vi "ISEG_HVSystem.constructor.vi"(0 "name":string, 2 "data in":string, 5 "error in (no error)":errorcluster) -> (14 "i ref out":refnum<vi>, 16 "data out":string, 19 "error out":errorcluster)   [LabVIEW 2014, in "ISEG_HVSystem.lvlib"]
doc: "This is the constructor of a class.\n\nLicense Agreement for this software:\n\nCopyright (C)\nGesellschaft für Schwerionenforschung, GSI\nPlanckstr. 1\n64291 Darmstadt\nGermany\n\nContact: D.Beck@gsi.de \n\nThis program is free software; you can redistribute it and/or modify it under the terms of the \nGNU General Public License as published by the Free Software Foundation; either version 2 of \nthe license, or (at your option) any later version.\n\nThis program is distributed in the hope that it will be useful, but WITHOUT ANY WARRANTY; \nwithout even the implied warranty of MERCHANTABILITY or FITNESS FOR A PARTICULAR PURPOSE. See the GNU General License for more details (http://www.gnu.org).\n\nGesellschaft für Schwerionenforschung, GSI\nPlanckstr. 1, 64291 Darmstadt, Germany\nFor all questions and ideas contact: M.Richter@gsi.de, H.Brand@gsi.de or D.Beck@gsi.de.\nLast update: 16-JUN-2004"
uses:
  ISEG_HVSystem.lvlib
  ISEG_HVSystem.i attribute.ctl
  ISEG_HVSystem.DIM Status.ctl
  CSCore/CSApplicationBaseClasses/DeviceBase/DeviceBase.myEventNames.ctl
  CSCore/CSApplicationBaseClasses/DeviceBase/DeviceBase.lvlib
  CSCore/CSSystem/CSSystemLib/CSSystemLib.lvlib
  CSCore/BaseProcess/BaseProcess.lvlib
panel:
  in  "CLASS.i attribute":T1
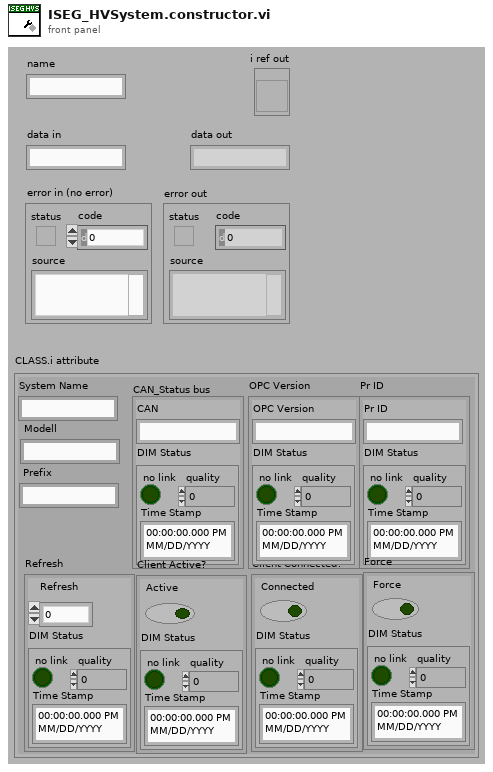
[diagram p1: front panel]
types:
  T1 = typedef "ISEG_HVSystem.lvlib/ISEG_HVSystem.i attribute.ctl" = cluster{"System Name":string, "CAN_Status bus":cluster{"CAN":string, "DIM Status":T2}, "Client Active?":cluster{"Active":bool, "DIM Status":T2}, "Client Connected?":cluster{"Connected":bool, "DIM Status":T2}, "OPC Version":cluster{"OPC Version":string, "DIM Status":T2}, "Pr ID":cluster{"Pr ID":string, "DIM Status":T2}, " Modell":string, " Prefix":string, "Force":cluster{"Force":bool, "DIM Status":T2}, "Refresh":cluster{"Refresh":dbl, "DIM Status":T2}}
  T2 = typedef "ISEG_HVSystem.lvlib/ISEG_HVSystem.DIM Status.ctl" = cluster{"no link":bool, "quality":i32, "Time Stamp":timestamp}
  T3 = enum16{"SetAttribute", "GetAttribute", "CreateAttribute", "DestroyAttribute", "DestroyAllAtributes"}
  T4 = typedef "DeviceBase.lvlib/DeviceBase.myEventNames.ctl" = enum16{"lvmsg://Initialize", "lvmsg://Close", "lvmsg://Configure", "lvmsg://Reset", "lvmsg://IDQuery"}
  T5 = typedef "BaseProcess.lvlib/BaseProcess.i attribute.ctl" = cluster{"EventStatus":string, "EventError":i32, "PresetEvtWatchD":i32, "PresetPdcWatchD":i32, "EventTimeout":i32, "PeriodicInterval":i32, "Interface":string[], "Address":string[], "Special":string[], "PeriodicError":i32, "PeriodicStatus":string, "SuperProc":string, "Descriptors":T6[], "CaseRef":refnum<vi>, "PdcRef":refnum<vi>, "Thread Ref":refnum<vi>, "eventErrorID":i32, "eventStatusID":i32, "periodicErrorID":i32, "periodicStatusID":i32, "pdcCtrID":i32}
  T6 = typedef "BaseProcess.lvlib/BaseProcess.descriptor definition.ctl" = cluster{"selector":string, "descriptor":T7}
  T7 = typedef "BaseProcess.lvlib/BaseProcess.descriptor string definition.ctl" = string
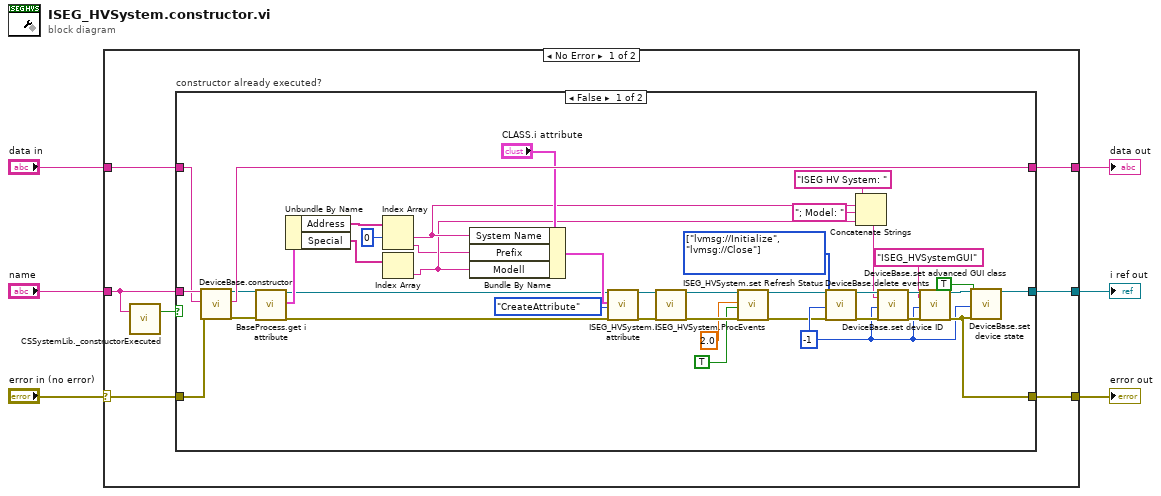
[diagram p0: block diagram]
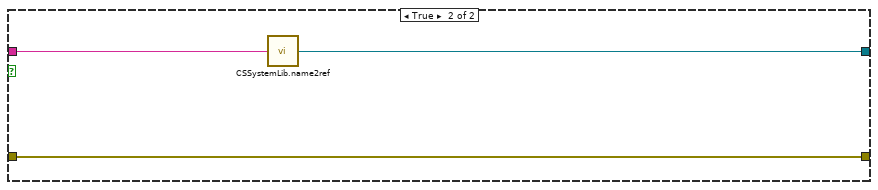
[diagram p2: hidden frame]
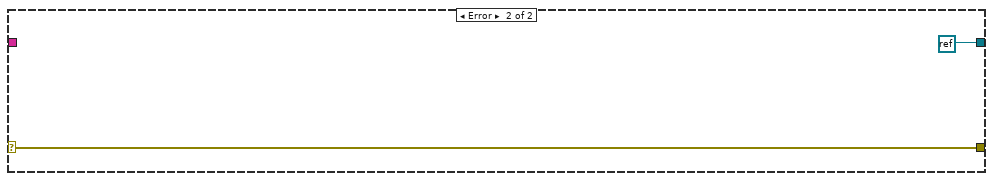
[diagram p3: hidden frame]
diagram:
  n1 = case shown="No Error" "error in (no error)" {
    selector: "error in (no error)" -> [w11 w57]
    tunnel: "name" -> [w10 _]
    tunnel: [w13 refnum<k0> refnum ("Not a Refnum Constant")] -> w5
    tunnel: [w12 w57] -> w4
    tunnel: "data in" -> [w8 _]
    tunnel: [w7 _] -> w1
    frame No Error {
      n2 = call "CSSystemLib._constructorExecuted.vi"("name"=w10) -> ("constructor executed?"=w9:bool)  [unwired: 18 in]
      n3 = case "constructor already executed?" shown="False" w9 {
        tunnel: w10 -> [w52 w56]
        tunnel: [w32 w55] -> w13
        tunnel: [w23 w54] -> w12
        tunnel: w11 -> [w49 w54]
        tunnel: w8 -> [w48 _]
        tunnel: [w46 _] -> w7
        frame False {
          w47 = T4[] [enum."lvmsg://Initialize", enum."lvmsg://Close"] items=["lvmsg://Initialize", "lvmsg://Close", "lvmsg://Configure", "lvmsg://Reset", "lvmsg://IDQuery"] ("events")
          w21 = -1 ("ms timeout (10000)")
          n4 = call "DeviceBase.constructor.vi"("name"=w52, "data in"=w48, "error in (no error)"=w49) -> ("i ref out"=w38:refnum<vi>, "data out"=w46:string, "error out"=w39:errorcluster)  [unwired: 14 in]
          n5 = call "BaseProcess.get i attribute.vi"("i ref in"=w38, "error in (no error)"=w39) -> ("i ref out"=w36:refnum<vi>, "i attribute"=w42:T5, "error out"=w37:errorcluster)  [unwired: 15 in]
          n6 = Unbundle By Name(w42) -> ("Address"=w45:string[], "Special"=w44:string[])
          n7 = Index Array(array=w45, index #1=0 ("index")) -> (element #1=w27:string, element #2=w20:string)  [unwired: 1 in]
          n8 = Index Array(array=w44) -> (element=w26:string)  [unwired: 1 in]
          n9 = Bundle By Name(cluster="CLASS.i attribute", "System Name"=w27, "Prefix"=w20, "Modell"=w26) -> (w40:T1)
          n10 = call "ISEG_HVSystem.i attribute.vi"("VI Refnum"=w36, "CLASS.i attribute"=w40, "Action"=T3."CreateAttribute", "error in (no error)"=w37) -> ("VI Refnum out"=w51:refnum<vi>, "error out"=w50:errorcluster)  [unwired: 13 in, 1 out]
          n11 = call "ISEG_HVSystem.ProcEvents.vi"("i ref in"=w51, "error in (no error)"=w50) -> ("i ref out"=w19:refnum<vi>, "error out"=w17:errorcluster)  [unwired: 16 in]
          n12 = call "ISEG_HVSystem.set Refresh Status.vi"("i ref in"=w19, "Refresh Status"=2.0, "Force"=TRUE, "error in (no error)"=w17) -> ("i ref out"=w18:refnum<vi>, "error out"=w16:errorcluster)  [unwired: 14 in]
          n13 = call "DeviceBase.delete events.vi"("i ref in"=w18, "events"=w47, "ms timeout (10000)"=w21, "error in (no error)"=w16) -> ("i ref out"=w31:refnum<vi>, "error out"=w30:errorcluster)  [unwired: 13 in, 1 out]
          n14 = Concatenate Strings("ISEG HV System: " ("string"), w27, "; Model: " ("string"), w26) -> (w25:string)
          n15 = call "DeviceBase.set device ID.vi"("i ref in"=w31, "deviceID"=w25, "ms timeout (10000)"=w21, "error in (no error)"=w30) -> ("i ref out"=w35:refnum<vi>, "error out"=w34:errorcluster)  [unwired: 13 in, 1 out]
          n16 = call "DeviceBase.set advanced GUI class.vi"("i ref in"=w35, "advancedGUIClass"="ISEG_HVSystemGUI", "ms timeout (10000)"=w21, "error in (no error)"=w34) -> ("i ref out"=w33:refnum<vi>, "error out"=w23:errorcluster)  [unwired: 13 in, 1 out]
          n17 = call "DeviceBase.set device state.vi"("i ref in"=w33, "implicit"=TRUE, "ms timeout (10000)"=w21, "error in (no error)"=w23) -> ("i ref out"=w32:refnum<vi>)  [unwired: 13 in, 2 out]
        }
        frame True {
          n18 = call "CSSystemLib.name2ref.vi"("name"=w56) -> ("obj refnum"=w55:refnum<vi>)
        }
      }
    }
    frame Error {
    }
  }
  "i ref out" <- w5
  "error out" <- w4
  "data out" <- w1
